vi "Main.vi"() -> ()   [LabVIEW 2018] (continued)
            n721 = Match Pattern(string=w6025, regular expression=w6022) -> (before substring=→"ST60 Sleeve 5020302":string)  [unwired: 1 in, 3 out]
            n722 = Match Pattern(string=w6024, regular expression=w6022) -> (before substring=→"ST60 Eclip 5018568":string)  [unwired: 1 in, 3 out]
            n723 = Match Pattern(string=w6023, regular expression=w6022) -> (before substring=→"ST70 Shaft Seal 5024366":string)  [unwired: 1 in, 3 out]
          }
        }
      }
      n724 = while {
        shift-right: [w4267] -> _
        shift-left: cluster{"Data":string[], "State":T1} {"Data"=[], "State"=enum."PLC通讯初始化"} ("元素") -> [w4268]
        shift-right: [w4276] -> _
        shift-left: w124 -> [w4273]
        shift-right: [w4277] -> _
        shift-left: _ -> [w4274]
        tunnel: w125 -> [w4269]
        tunnel: w123 -> [w4264]
        shift-right: [w4262] -> _
        shift-left: _ -> [w4263]
        tunnel: w122 -> [_]
        stop <- w4265 stop-if-true
        # "OP30"
        n725 = local read "退出"() -> (w4272:bool)
        n726 = Wait (ms)(milliseconds to wait=u32 20 ("等待时间（毫秒）")) -> ()  [unwired: 1 out]
        n727 = call "状态判断.vi"("error IO"=w4273, "退出？"=w4272, "簇 输入"=w4268, "队列输入"=w4269) -> ("簇"=w4271:cluster{"Data":string[], "State":T1})  [unwired: 6 in, 1 out]
        n728 = Unbundle By Name(w4271) -> ("Data"=w4266:string[], "State"=w4270:T1)
        "30_State" <- w4270
        n729 = case shown="\"读数据保存请求2\"" w4270 {
          tunnel: [w4287 w4326 w4346 w4377 w4398 w4450 w4470 w4516 w4529 w4544 w4564 w4609 w4628 w4682 w4688 w4752 w4779 w4795 refnum<k5> refnum ("TCP") refnum<k5> refnum ("TCP") w4814] -> w4277
          tunnel: [w4288 errorcluster {"status"=FALSE, "code"=0, "source"=""} ("error out") w4345 w4373 w4397 errorcluster {"status"=FALSE, "code"=0, "source"=""} ("error out") w4469 w4496 w4530 errorcluster {"status"=FALSE, "code"=0, "source"=""} ("error out") w4565 w4606 w4627 errorcluster {"status"=FALSE, "code"=0, "source"=""} ("error out") w4687 w4748 w4780 errorcluster {"status"=FALSE, "code"=0, "source"=""} ("error out") errorcluster {"status"=FALSE, "code"=0, "source"=""} ("error out") w4808 w4815] -> w4276
          tunnel: w4274 -> [_ w4326 w4347 w4378 w4399 w4450 w4471 w4498 w4532 w4544 w4550 w4611 w4632 w4682 w4690 w4742 w4783 w4795 w4802 w4809 w4826]
          tunnel: w4269 -> [w4317 _ w4328 _ _ _ w4451 _ _ _ w4562 _ _ _ w4686 _ _ _ w4798 w4810 _]
          tunnel: [cluster{"Data":string[], "State":T1} {"Data"=[], "State"=enum."读扫码请求"} ("元素") cluster{"Data":string[], "State":T1} {"Data"=[], "State"=enum."读扫码请求"} ("元素") w4335 cluster{"Data":string[], "State":T1} {"Data"=[], "State"=enum."读数据保存请求"} ("元素") cluster{"Data":string[], "State":T1} {"Data"=[], "State"=enum."读数据保存请求"} ("元素") cluster{"Data":string[], "State":T1} {"Data"=[], "State"=enum."读数据保存请求"} ("元素") w4459 cluster{"Data":string[], "State":T1} {"Data"=[], "State"=enum."读扫码请求2"} ("元素") cluster{"Data":string[], "State":T1} {"Data"=[], "State"=enum."读扫码请求2"} ("元素") cluster{"Data":string[], "State":T1} {"Data"=[], "State"=enum."读扫码请求2"} ("元素") w4563 cluster{"Data":string[], "State":T1} {"Data"=[], "State"=enum."读数据保存请求2"} ("元素") cluster{"Data":string[], "State":T1} {"Data"=[], "State"=enum."读数据保存请求2"} ("元素") cluster{"Data":string[], "State":T1} {"Data"=[], "State"=enum."读数据保存请求2"} ("元素") w4684 cluster{"Data":string[], "State":T1} {"Data"=[], "State"=enum."看门狗"} ("元素") cluster{"Data":string[], "State":T1} {"Data"=[], "State"=enum."看门狗"} ("元素") cluster{"Data":string[], "State":T1} {"Data"=[], "State"=enum."看门狗"} ("元素") cluster{"Data":string[], "State":T1} {"Data"=[], "State"=enum."PLC通讯初始化"} ("元素") cluster{"Data":string[], "State":T1} {"Data"=[], "State"=enum."退出"} ("元素") cluster{"Data":string[], "State":T1} {"Data"=[], "State"=enum."读扫码请求"} ("元素")] -> w4267
          tunnel: w4266 -> [_ _ _ _ w4396 _ _ _ w4531 _ _ _ w4631 _ _ _ w4781 _ _ _ _]
          tunnel: [FALSE FALSE FALSE FALSE FALSE FALSE FALSE FALSE FALSE FALSE FALSE FALSE FALSE FALSE FALSE FALSE FALSE FALSE FALSE TRUE FALSE] -> w4265
          tunnel: w4264 -> [_ _ _ _ _ _ _ w4508 _ _ _ _ _ _ _ _ _ _ w4799 w4811 _]
          tunnel: w4263 -> [_ w4322 w4329 w4374 w4394 w4446 w4452 w4499 w4526 w4540 w4549 w4610 w4633 w4683 w4689 w4750 w4782 w4796 w4797 w4806 w4819]
          tunnel: [T8 {"扫码2超时"="999", "扫码1超时"="999", "数据保存1超时"="999", "看门狗"="0", "数据保存2超时"="999"} w4322 w4329 w4374 w4393 w4446 w4452 w4499 w4524 w4540 w4548 w4610 w4626 w4683 w4689 w4750 w4777 w4796 w4797 w4806 w4818] -> w4262
          frame "PLC通讯初始化", Default {
            w4301 = u16 0 items=["byte", "word", "Dword"] ("数据类型")
            w4305 = u8 132 items=["I/O (P)"=128, "Input (I)"=129, "Output (Q)"=130, "Bit Memory (M)"=131, "Data (DB)"=132, "Instance Data (DI)"=133, "Local Data (L)"=134, "Predecessor Local Data (VL)"=135] ("寄存器类型")
            w4296 = u16 0 items=["byte", "word", "Dword"] ("数据类型")
            w4292 = u8 132 items=["I/O (P)"=128, "Input (I)"=129, "Output (Q)"=130, "Bit Memory (M)"=131, "Data (DB)"=132, "Instance Data (DI)"=133, "Local Data (L)"=134, "Predecessor Local Data (VL)"=135] ("寄存器类型")
            w4320 = u8 0 items=["S7-1200.200.200SMART"=0, "S7-300"=2, "S7-400"=3] ("PLC 系列")
            n730 = Enqueue Element(queue=w4317, element=cluster{"Data":string[], "State":T1} {"Data"=["999"], "State"=enum."扫码回复"} ("元素")) -> (queue out=w4313:refnum<queue>, error out=w4312:errorcluster)  [unwired: 2 in, 1 out]
            n731 = call "S7_Open.vi"("IP 地址"="192.168.0.30", "PLC 系列"=w4320, "超时（MS）"=100) -> ("TCP"=w4291:refnum<k5>, "error out"=w4290:errorcluster)  [unwired: 10 in, 1 out]
            n732 = Enqueue Element(queue=w4313, element=cluster{"Data":string[], "State":T1} {"Data"=["999"], "State"=enum."扫码回复2"} ("元素"), error in (no error)=w4312) -> (queue out=w4311:refnum<queue>, error out=w4310:errorcluster)  [unwired: 1 in, 1 out]
            n733 = Unbundle By Name(w4290) -> ("status"=→"ST30通讯状态":bool)
            n734 = call "S7_Read.vi"("TCP"=w4291, "DB #"=u16 20, "读取长度"=u16 17, "寄存器类型"=w4292, "起始地址"=u32 24, "数据类型"=w4296, "error in"=w4290) -> ("TCP"=w4306:refnum<k5>, "数据"=w4297:u32[], "error out"=w4289:errorcluster)  [unwired: 5 in, 1 out]
            n735 = Enqueue Element(queue=w4311, element=cluster{"Data":string[], "State":T1} {"Data"=["999"], "State"=enum."数据保存回复"} ("元素"), error in (no error)=w4310) -> (queue out=w4285:refnum<queue>, error out=w4284:errorcluster)  [unwired: 1 in, 1 out]
            n736 = To Unsigned Word Integer(number=w4297) -> (unsigned 16bit integer=w4298:u16[])
            n737 = call "还原为字符串.vi"("输入数组"=w4298) -> ("字符串"=w4282:string)  [unwired: 9 in, 1 out]
            n738 = Match Pattern(string=w4282, regular expression=" " ("正则表达式")) -> (before substring=w4281:string)  [unwired: 1 in, 3 out]
            n739 = local write "301 二维码"(w4281) -> ()
            n740 = Enqueue Element(queue=w4285, element=cluster{"Data":string[], "State":T1} {"Data"=["999"], "State"=enum."数据保存回复2"} ("元素"), error in (no error)=w4284) -> ()  [unwired: 1 in, 3 out]
            n741 = call "S7_Read.vi"("TCP"=w4306, "DB #"=u16 20, "读取长度"=u16 17, "寄存器类型"=w4305, "起始地址"=u32 42, "数据类型"=w4301, "error in"=w4289) -> ("TCP"=w4287:refnum<k5>, "数据"=w4300:u32[], "error out"=w4288:errorcluster)  [unwired: 5 in, 1 out]
            n742 = To Unsigned Word Integer(number=w4300) -> (unsigned 16bit integer=w4299:u16[])
            n743 = call "还原为字符串.vi"("输入数组"=w4299) -> ("字符串"=w4279:string)  [unwired: 9 in, 1 out]
            n744 = Match Pattern(string=w4279, regular expression=" " ("正则表达式")) -> (before substring=w4278:string)  [unwired: 1 in, 3 out]
            n745 = local write "302 二维码"(w4278) -> ()
          }
          frame "---------------" {
          }
          frame "读扫码请求" {
            w4355 = u16 0 items=["byte", "word", "Dword"] ("数据类型")
            w4357 = u8 132 items=["I/O (P)"=128, "Input (I)"=129, "Output (Q)"=130, "Bit Memory (M)"=131, "Data (DB)"=132, "Instance Data (DI)"=133, "Local Data (L)"=134, "Predecessor Local Data (VL)"=135] ("寄存器类型")
            n746 = call "S7_Read.vi"("TCP"=w4347, "DB #"=u16 20, "读取长度"=u16 1, "寄存器类型"=w4357, "起始地址"=u32 0, "数据类型"=w4355) -> ("TCP"=w4346:refnum<k5>, "数据"=w4352:u32[], "error out"=w4345:errorcluster)  [unwired: 6 in, 1 out]
            n747 = Index Array(array=w4352, index=0 ("索引")) -> (element=w4350:u32)
            n748 = Number To Boolean Array(number=w4350) -> (Boolean array=w4349:bool[])
            n749 = Index Array(array=w4349, index=0 ("索引")) -> (element=w4327:bool)
            "ST301扫码请求" <- w4327
            n750 = Unbundle By Name(w4329) -> ("扫码1超时"=w4330:string)
            n751 = Not Equal?(x=w4330, y="999") -> (x != y?=w4332:bool)
            n752 = Not(x=w4332) -> (.not. x?=w4333:bool)
            n753 = call <vilib>:"Boolean Crossing PtByPt.vi"("direction"=enum16{"either", "false-true", "true-false"}."false-true", "input"=w4327) -> ("crossing"=w4341:bool)  [unwired: 1 in]
            n754 = call <vilib>:"Boolean Crossing PtByPt.vi"("direction"=enum16{"either", "false-true", "true-false"}."true-false", "input"=w4327) -> ("crossing"=w4340:bool)  [unwired: 1 in]
            n755 = call "已用时间7"("Reset"=w4333) -> ("Time has Elapsed"=w4334:bool)  [unwired: 11 in, 7 out]
            n756 = Insert Into Array(array=bool[] [] ("数组"), index=0 ("索引"), new element #1=w4341, new element #2=w4340) -> (w4337:bool[])
            n757 = Boolean Array To Number(Boolean array=w4337) -> (number=w4336:u32)
            n758 = case shown="0, 默认" w4336 {
              tunnel: [cluster{"Data":string[], "State":T1} {"Data"=[], "State"=enum."读数据保存请求"} ("元素") w4363 w4366] -> w4335
              tunnel: w4328 -> [_ w4364 w4367]
              frame 0, Default {
              }
              frame 1 {
                w4363 = cluster{"Data":string[], "State":T1} {"Data"=[], "State"=enum."读二维码"} ("元素")
                n759 = Enqueue Element(queue=w4364, element=w4363, timeout in ms (-1)=10 ("超时毫秒(-1)")) -> ()  [unwired: 1 in, 3 out]
              }
              frame 2 {
                w4366 = cluster{"Data":string[], "State":T1} {"Data"=["999"], "State"=enum."扫码回复"} ("元素")
                n760 = Enqueue Element(queue=w4367, element=w4366, timeout in ms (-1)=10 ("超时毫秒(-1)")) -> ()  [unwired: 1 in, 3 out]
              }
            }
            n761 = case shown="真" w4334 {
              tunnel: w4328 -> [_ w4359]
              frame False {
              }
              frame True {
                n762 = Enqueue Element(queue=w4359, element=cluster{"Data":string[], "State":T1} {"Data"=["999"], "State"=enum."扫码回复"} ("元素"), timeout in ms (-1)=10 ("超时毫秒(-1)")) -> ()  [unwired: 1 in, 3 out]
              }
            }
          }
          frame "读二维码" {
            w4383 = u16 0 items=["byte", "word", "Dword"] ("数据类型")
            w4379 = u8 132 items=["I/O (P)"=128, "Input (I)"=129, "Output (Q)"=130, "Bit Memory (M)"=131, "Data (DB)"=132, "Instance Data (DI)"=133, "Local Data (L)"=134, "Predecessor Local Data (VL)"=135] ("寄存器类型")
            n763 = call "S7_Read.vi"("TCP"=w4378, "DB #"=u16 20, "读取长度"=u16 17, "寄存器类型"=w4379, "起始地址"=u32 24, "数据类型"=w4383) -> ("TCP"=w4377:refnum<k5>, "数据"=w4384:u32[], "error out"=w4386:errorcluster)  [unwired: 6 in, 1 out]
            n764 = To Unsigned Word Integer(number=w4384) -> (unsigned 16bit integer=w4385:u16[])
            n765 = call "还原为字符串.vi"("error in (no error)"=w4386, "输入数组"=w4385) -> ("error out"=w4370:errorcluster, "字符串"=w4371:string)  [unwired: 8 in]
            n766 = Match Pattern(string=w4371, regular expression=" " ("正则表达式")) -> (before substring=w4368:string)  [unwired: 1 in, 3 out]
            n767 = flat-sequence {
              tunnel: w4370 -> [w4388]
              tunnel: [w4388] -> w4369
              tunnel: w4368 -> [w4387]
              tunnel: [w4390] -> w4373
              tunnel: w4369 -> [w4389]
              frame #0 {
                "301 二维码" <- w4387
              }
              frame #1 {
                n768 = property on="ST301扫码请求 (事件)" class="Bool (严格)"(error in=w4389, "Val(Sgnl)"=TRUE ("值(信号)")) -> (error out=w4390:errorcluster)  [unwired: 1 in, 1 out]
              }
            }
          }
          frame "扫码回复" {
            n769 = Array Size(array=w4396) -> (size(s)=w4395:i32)
            n770 = case shown="1" w4395 {
              tunnel: w4399 -> [w4414 w4437]
              tunnel: [w4405 w4439] -> w4398
              tunnel: [w4404 w4438] -> w4397
              tunnel: w4396 -> [w4403 w4436]
              tunnel: [w4402 w4434] -> w4392
              frame 3, Default {
                w4417 = u8 132 items=["I/O (P)"=128, "Input (I)"=129, "Output (Q)"=130, "Bit Memory (M)"=131, "Data (DB)"=132, "Instance Data (DI)"=133, "Local Data (L)"=134, "Predecessor Local Data (VL)"=135] ("寄存器类型")
                w4416 = u16 1 items=["byte", "word", "Dword"] ("数据类型")
                w4424 = u8 132 items=["I/O (P)"=128, "Input (I)"=129, "Output (Q)"=130, "Bit Memory (M)"=131, "Data (DB)"=132, "Instance Data (DI)"=133, "Local Data (L)"=134, "Predecessor Local Data (VL)"=135] ("寄存器类型")
                w4425 = u16 1 items=["byte", "word", "Dword"] ("数据类型")
                w4430 = u8 132 items=["I/O (P)"=128, "Input (I)"=129, "Output (Q)"=130, "Bit Memory (M)"=131, "Data (DB)"=132, "Instance Data (DI)"=133, "Local Data (L)"=134, "Predecessor Local Data (VL)"=135] ("寄存器类型")
                w4429 = u16 1 items=["byte", "word", "Dword"] ("数据类型")
                n771 = Index Array(array=w4403) -> (element #1=w4402:string, element #2=w4410:string, element #3=w4409:string)  [unwired: 3 in]
                n772 = Equal?(x=w4409, y="OK") -> (x = y?=w4407:bool)
                n773 = Decimal String To Number(string=w4410, default (0L)=u32 0 ("默认(0 I32)")) -> (number=w4411:u32)  [unwired: 1 in, 1 out]
                n774 = case shown="真" w4407 {
                  tunnel: [u32 2 ("写入数据") u32 1 ("写入数据")] -> w4406
                  frame False {
                  }
                  frame True {
                  }
                }
                n775 = call "S7_Write.vi"("TCP"=w4414, "寄存器类型"=w4430, "DB #"=u16 20, "写入地址"=u32 8, "数据类型"=w4429, "写入数据"=w4411) -> ("TCP"=w4421:refnum<k5>, "error out"=w4422:errorcluster)  [unwired: 7 in, 1 out]
                n776 = call "S7_Write.vi"("TCP"=w4421, "寄存器类型"=w4424, "DB #"=u16 20, "写入地址"=u32 10, "数据类型"=w4425, "写入数据"=w4406, "error in"=w4422) -> ("TCP"=w4413:refnum<k5>, "error out"=w4412:errorcluster)  [unwired: 6 in, 1 out]
                n777 = Decimal String To Number(string=w4402, default (0L)=u32 0 ("默认(0 I32)")) -> (number=w4420:u32)  [unwired: 1 in, 1 out]
                n778 = call "S7_Write.vi"("TCP"=w4413, "寄存器类型"=w4417, "DB #"=u16 20, "写入地址"=u32 2, "数据类型"=w4416, "写入数据"=w4420, "error in"=w4412) -> ("TCP"=w4405:refnum<k5>, "error out"=w4404:errorcluster)  [unwired: 6 in, 1 out]
              }
              frame 1 {
                w4442 = u8 132 items=["I/O (P)"=128, "Input (I)"=129, "Output (Q)"=130, "Bit Memory (M)"=131, "Data (DB)"=132, "Instance Data (DI)"=133, "Local Data (L)"=134, "Predecessor Local Data (VL)"=135] ("寄存器类型")
                w4441 = u16 1 items=["byte", "word", "Dword"] ("数据类型")
                n779 = Index Array(array=w4436, index=0 ("索引")) -> (element=w4434:string)
                n780 = Decimal String To Number(string=w4434, default (0L)=u32 0 ("默认(0 I32)")) -> (number=w4445:u32)  [unwired: 1 in, 1 out]
                n781 = call "S7_Write.vi"("TCP"=w4437, "寄存器类型"=w4442, "DB #"=u16 20, "写入地址"=u32 2, "数据类型"=w4441, "写入数据"=w4445) -> ("TCP"=w4439:refnum<k5>, "error out"=w4438:errorcluster)  [unwired: 7 in, 1 out]
              }
            }
            "扫码请求回复301" <- w4392
            n782 = Bundle By Name(cluster=w4394, "扫码1超时"=w4392) -> (w4393:T8)
          }
          frame "-------------" {
          }
          frame "读数据保存请求" {
            w4479 = u16 0 items=["byte", "word", "Dword"] ("数据类型")
            w4481 = u8 132 items=["I/O (P)"=128, "Input (I)"=129, "Output (Q)"=130, "Bit Memory (M)"=131, "Data (DB)"=132, "Instance Data (DI)"=133, "Local Data (L)"=134, "Predecessor Local Data (VL)"=135] ("寄存器类型")
            n783 = call "S7_Read.vi"("TCP"=w4471, "DB #"=u16 20, "读取长度"=u16 1, "寄存器类型"=w4481, "起始地址"=u32 0, "数据类型"=w4479) -> ("TCP"=w4470:refnum<k5>, "数据"=w4476:u32[], "error out"=w4469:errorcluster)  [unwired: 6 in, 1 out]
            n784 = Index Array(array=w4476, index=0 ("索引")) -> (element=w4474:u32)
            n785 = Number To Boolean Array(number=w4474) -> (Boolean array=w4473:bool[])
            n786 = Unbundle By Name(w4452) -> ("数据保存1超时"=w4453:string)
            n787 = Index Array(array=w4473, index=1 ("索引")) -> (element=w4458:bool)
            "ST301数据读取" <- w4458
            n788 = Not Equal?(x=w4453, y="999") -> (x != y?=w4455:bool)
            n789 = Not(x=w4455) -> (.not. x?=w4456:bool)
            n790 = call <vilib>:"Boolean Crossing PtByPt.vi"("direction"=enum16{"either", "false-true", "true-false"}."false-true", "input"=w4458) -> ("crossing"=w4462:bool)  [unwired: 1 in]
            n791 = call <vilib>:"Boolean Crossing PtByPt.vi"("direction"=enum16{"either", "false-true", "true-false"}."true-false", "input"=w4458) -> ("crossing"=w4463:bool)  [unwired: 1 in]
            n792 = call "已用时间8"("Reset"=w4456) -> ("Time has Elapsed"=w4457:bool)  [unwired: 11 in, 7 out]
            n793 = Insert Into Array(array=bool[] [] ("数组"), index=0 ("索引"), new element #1=w4462, new element #2=w4463) -> (w4466:bool[])
            n794 = Boolean Array To Number(Boolean array=w4466) -> (number=w4467:u32)
            n795 = case shown="2" w4467 {
              tunnel: [cluster{"Data":string[], "State":T1} {"Data"=[], "State"=enum."读扫码请求2"} ("元素") w4487 w4489] -> w4459
              tunnel: w4451 -> [_ w4488 w4490]
              frame 0, Default {
              }
              frame 1 {
                w4487 = cluster{"Data":string[], "State":T1} {"Data"=[], "State"=enum."读数据"} ("元素")
                n796 = Enqueue Element(queue=w4488, element=w4487, timeout in ms (-1)=10 ("超时毫秒(-1)")) -> ()  [unwired: 1 in, 3 out]
              }
              frame 2 {
                w4489 = cluster{"Data":string[], "State":T1} {"Data"=["999"], "State"=enum."数据保存回复"} ("元素")
                n797 = Enqueue Element(queue=w4490, element=w4489, timeout in ms (-1)=10 ("超时毫秒(-1)")) -> ()  [unwired: 1 in, 3 out]
              }
            }
            n798 = case shown="真" w4457 {
              tunnel: w4451 -> [_ w4483]
              frame False {
              }
              frame True {
                n799 = Enqueue Element(queue=w4483, element=cluster{"Data":string[], "State":T1} {"Data"=["999"], "State"=enum."数据保存回复"} ("元素"), timeout in ms (-1)=10 ("超时毫秒(-1)")) -> ()  [unwired: 1 in, 3 out]
              }
            }
          }
          frame "读数据" {
            w4517 = u16 1 items=["byte", "word", "Dword"] ("数据类型")
            w4521 = u8 132 items=["I/O (P)"=128, "Input (I)"=129, "Output (Q)"=130, "Bit Memory (M)"=131, "Data (DB)"=132, "Instance Data (DI)"=133, "Local Data (L)"=134, "Predecessor Local Data (VL)"=135] ("寄存器类型")
            n800 = call "S7_Read.vi"("TCP"=w4498, "DB #"=u16 20, "读取长度"=u16 1, "寄存器类型"=w4521, "起始地址"=u32 6, "数据类型"=w4517) -> ("TCP"=w4516:refnum<k5>, "数据"=w4513:u32[], "error out"=w4507:errorcluster)  [unwired: 6 in, 1 out]
            n801 = local read "ST301 Dowel Pin 5024533"() -> (w4493:string)
            n802 = local read "ST301 Dowel Pin 5020282"() -> (w4492:string)
            n803 = Index Array(array=w4513) -> (element=w4512:u32)  [unwired: 1 in]
            n804 = local read "ST301 Vane 5004737"() -> (w4494:string)
            n805 = Equal?(x=w4512, y=u32 1) -> (x = y?=w4510:bool)
            n806 = case shown="真" w4510 {
              tunnel: ["NG" "OK"] -> w4500
              frame False {
              }
              frame True {
              }
            }
            n807 = Format Date/Time String(time format string (%c)="%Y-%m-%d" ("时间格式字符串(%c)")) -> (date/time string=w4502:string)  [unwired: 2 in]
            n808 = Get Date/Time String() -> (time string=w4501:string)  [unwired: 3 in, 1 out]
            n809 = Insert Into Array(array=string[] [] ("数组"), index=0 ("索引"), new element #1="301" ("新元素/子数组"), new element #2=w4500, new element #3=w4502, new element #4=w4501, new element #5=w4500, new element #6=w4494, new element #7=w4493, new element #8=w4492) -> (w4509:string[])
            n810 = Enqueue Element(queue=w4508, element=w4509, error in (no error)=w4507) -> (error out=w4497:errorcluster)  [unwired: 1 in, 2 out]
            n811 = property on="ST301数据读取 (事件)" class="Bool (严格)"(error in=w4497, "Val(Sgnl)"=TRUE ("值(信号)")) -> (error out=w4496:errorcluster)  [unwired: 1 in, 1 out]
          }
          frame "数据保存回复" {
            w4537 = u8 132 items=["I/O (P)"=128, "Input (I)"=129, "Output (Q)"=130, "Bit Memory (M)"=131, "Data (DB)"=132, "Instance Data (DI)"=133, "Local Data (L)"=134, "Predecessor Local Data (VL)"=135] ("寄存器类型")
            w4538 = u16 1 items=["byte", "word", "Dword"] ("数据类型")
            n812 = Index Array(array=w4531, index=0 ("索引")) -> (element=w4525:string)
            "数据保存请求回复301" <- w4525
            n813 = Decimal String To Number(string=w4525, default (0L)=u32 0 ("默认(0 I32)")) -> (number=w4533:u32)  [unwired: 1 in, 1 out]
            n814 = call "S7_Write.vi"("TCP"=w4532, "寄存器类型"=w4537, "DB #"=u16 20, "写入地址"=u32 4, "数据类型"=w4538, "写入数据"=w4533) -> ("TCP"=w4529:refnum<k5>, "error out"=w4530:errorcluster)  [unwired: 7 in, 1 out]
            n815 = Bundle By Name(cluster=w4526, "数据保存1超时"=w4525) -> (w4524:T8)
          }
          frame "-----------------" {
          }
          frame "读扫码请求2" {
            w4558 = u8 132 items=["I/O (P)"=128, "Input (I)"=129, "Output (Q)"=130, "Bit Memory (M)"=131, "Data (DB)"=132, "Instance Data (DI)"=133, "Local Data (L)"=134, "Predecessor Local Data (VL)"=135] ("寄存器类型")
            w4557 = u16 1 items=["byte", "word", "Dword"] ("数据类型")
            w4566 = u16 0 items=["byte", "word", "Dword"] ("数据类型")
            w4568 = u8 132 items=["I/O (P)"=128, "Input (I)"=129, "Output (Q)"=130, "Bit Memory (M)"=131, "Data (DB)"=132, "Instance Data (DI)"=133, "Local Data (L)"=134, "Predecessor Local Data (VL)"=135] ("寄存器类型")
            n816 = Unbundle By Name(w4549) -> ("看门狗"=w4555:string)
            n817 = Decimal String To Number(string=w4555) -> (number=w4554:i32)  [unwired: 2 in, 1 out]
            n818 = Equal?(x=w4554, y=0) -> (x = y?=w4552:bool)
            n819 = case shown="假" w4552 {
              tunnel: [0 ("y") 1 ("y")] -> w4545
              frame False {
              }
              frame True {
              }
            }
            n820 = call "S7_Write.vi"("TCP"=w4550, "寄存器类型"=w4558, "DB #"=u16 20, "写入地址"=u32 22, "数据类型"=w4557, "写入数据"=w4545) -> ("TCP"=w4546:refnum<k5>, "error out"=w4547:errorcluster)  [unwired: 7 in, 1 out]
            n821 = Number To Decimal String(number=w4545) -> (decimal integer string=w4551:string)  [unwired: 1 in]
            n822 = local write "30"(w4545) -> ()
            n823 = Bundle By Name(cluster=w4549, "看门狗"=w4551) -> (w4548:T8)
            n824 = call "S7_Read.vi"("TCP"=w4546, "DB #"=u16 20, "读取长度"=u16 1, "寄存器类型"=w4568, "起始地址"=u32 0, "数据类型"=w4566, "error in"=w4547) -> ("TCP"=w4564:refnum<k5>, "数据"=w4588:u32[], "error out"=w4565:errorcluster)  [unwired: 5 in, 1 out]
            n825 = Index Array(array=w4588, index=0 ("索引")) -> (element=w4587:u32)
            n826 = Number To Boolean Array(number=w4587) -> (Boolean array=w4586:bool[])
            n827 = Index Array(array=w4586, index=2 ("索引")) -> (element=w4561:bool)
            "ST302扫码请求" <- w4561
            n828 = Unbundle By Name(w4548) -> ("扫码2超时"=w4578:string)
            n829 = Not Equal?(x=w4578, y="999") -> (x != y?=w4579:bool)
            n830 = Not(x=w4579) -> (.not. x?=w4580:bool)
            n831 = call <vilib>:"Boolean Crossing PtByPt.vi"("direction"=enum16{"either", "false-true", "true-false"}."false-true", "input"=w4561) -> ("crossing"=w4585:bool)  [unwired: 1 in]
            n832 = call <vilib>:"Boolean Crossing PtByPt.vi"("direction"=enum16{"either", "false-true", "true-false"}."true-false", "input"=w4561) -> ("crossing"=w4584:bool)  [unwired: 1 in]
            n833 = call "已用时间23"("Reset"=w4580) -> ("Time has Elapsed"=w4581:bool)  [unwired: 11 in, 7 out]
            n834 = Insert Into Array(array=bool[] [] ("数组"), index=0 ("索引"), new element #1=w4585, new element #2=w4584) -> (w4583:bool[])
            n835 = Boolean Array To Number(Boolean array=w4583) -> (number=w4582:u32)
            n836 = case shown="0, 默认" w4582 {
              tunnel: [cluster{"Data":string[], "State":T1} {"Data"=[], "State"=enum."读数据保存请求2"} ("元素") w4596 w4599] -> w4563
              tunnel: w4562 -> [_ w4597 w4600]
              frame 0, Default {
              }
              frame 1 {
                w4596 = cluster{"Data":string[], "State":T1} {"Data"=[], "State"=enum."读二维码2"} ("元素")
                n837 = Enqueue Element(queue=w4597, element=w4596, timeout in ms (-1)=10 ("超时毫秒(-1)")) -> ()  [unwired: 1 in, 3 out]
              }
              frame 2 {
                w4599 = cluster{"Data":string[], "State":T1} {"Data"=["999"], "State"=enum."扫码回复2"} ("元素")
                n838 = Enqueue Element(queue=w4600, element=w4599, timeout in ms (-1)=10 ("超时毫秒(-1)")) -> ()  [unwired: 1 in, 3 out]
              }
            }
            n839 = case shown="真" w4581 {
              tunnel: w4562 -> [_ w4592]
              frame False {
              }
              frame True {
                n840 = Enqueue Element(queue=w4592, element=cluster{"Data":string[], "State":T1} {"Data"=["999"], "State"=enum."扫码回复2"} ("元素"), timeout in ms (-1)=10 ("超时毫秒(-1)")) -> ()  [unwired: 1 in, 3 out]
              }
            }
          }
          frame "读二维码2" {
            w4612 = u16 0 items=["byte", "word", "Dword"] ("数据类型")
            w4614 = u8 132 items=["I/O (P)"=128, "Input (I)"=129, "Output (Q)"=130, "Bit Memory (M)"=131, "Data (DB)"=132, "Instance Data (DI)"=133, "Local Data (L)"=134, "Predecessor Local Data (VL)"=135] ("寄存器类型")
            n841 = call "S7_Read.vi"("TCP"=w4611, "DB #"=u16 20, "读取长度"=u16 17, "寄存器类型"=w4614, "起始地址"=u32 42, "数据类型"=w4612) -> ("TCP"=w4609:refnum<k5>, "数据"=w4617:u32[], "error out"=w4619:errorcluster)  [unwired: 6 in, 1 out]
            n842 = To Unsigned Word Integer(number=w4617) -> (unsigned 16bit integer=w4618:u16[])
            n843 = call "还原为字符串.vi"("error in (no error)"=w4619, "输入数组"=w4618) -> ("error out"=w4603:errorcluster, "字符串"=w4604:string)  [unwired: 8 in]
            n844 = Match Pattern(string=w4604, regular expression=" " ("正则表达式")) -> (before substring=w4601:string)  [unwired: 1 in, 3 out]
            n845 = flat-sequence {
              tunnel: w4603 -> [w4621]
              tunnel: [w4621] -> w4602
              tunnel: w4601 -> [w4620]
              tunnel: [w4623] -> w4606
              tunnel: w4602 -> [w4622]
              frame #0 {
                "302 二维码" <- w4620
              }
              frame #1 {
                n846 = property on="ST302扫码请求 (事件)" class="Bool (严格)"(error in=w4622, "Val(Sgnl)"=TRUE ("值(信号)")) -> (error out=w4623:errorcluster)  [unwired: 1 in, 1 out]
              }
            }
          }
          frame "扫码回复2" {
            n847 = Array Size(array=w4631) -> (size(s)=w4634:i32)
            n848 = case shown="1" w4634 {
              tunnel: w4632 -> [w4647 w4670]
              tunnel: [w4638 w4672] -> w4628
              tunnel: [w4637 w4671] -> w4627
              tunnel: w4631 -> [w4636 w4669]
              tunnel: [w4635 w4667] -> w4629
              frame 3, Default {
                w4650 = u8 132 items=["I/O (P)"=128, "Input (I)"=129, "Output (Q)"=130, "Bit Memory (M)"=131, "Data (DB)"=132, "Instance Data (DI)"=133, "Local Data (L)"=134, "Predecessor Local Data (VL)"=135] ("寄存器类型")
                w4649 = u16 1 items=["byte", "word", "Dword"] ("数据类型")
                w4657 = u8 132 items=["I/O (P)"=128, "Input (I)"=129, "Output (Q)"=130, "Bit Memory (M)"=131, "Data (DB)"=132, "Instance Data (DI)"=133, "Local Data (L)"=134, "Predecessor Local Data (VL)"=135] ("寄存器类型")
                w4658 = u16 1 items=["byte", "word", "Dword"] ("数据类型")
                w4663 = u8 132 items=["I/O (P)"=128, "Input (I)"=129, "Output (Q)"=130, "Bit Memory (M)"=131, "Data (DB)"=132, "Instance Data (DI)"=133, "Local Data (L)"=134, "Predecessor Local Data (VL)"=135] ("寄存器类型")
                w4662 = u16 1 items=["byte", "word", "Dword"] ("数据类型")
                n849 = Index Array(array=w4636) -> (element #1=w4635:string, element #2=w4643:string, element #3=w4642:string)  [unwired: 3 in]
                n850 = Equal?(x=w4642, y="OK") -> (x = y?=w4640:bool)
                n851 = Decimal String To Number(string=w4643, default (0L)=u32 0 ("默认(0 I32)")) -> (number=w4644:u32)  [unwired: 1 in, 1 out]
                n852 = case shown="真" w4640 {
                  tunnel: [u32 2 ("写入数据") u32 1 ("写入数据")] -> w4639
                  frame False {
                  }
                  frame True {
                  }
                }
                n853 = call "S7_Write.vi"("TCP"=w4647, "寄存器类型"=w4663, "DB #"=u16 20, "写入地址"=u32 18, "数据类型"=w4662, "写入数据"=w4644) -> ("TCP"=w4654:refnum<k5>, "error out"=w4655:errorcluster)  [unwired: 7 in, 1 out]
                n854 = call "S7_Write.vi"("TCP"=w4654, "寄存器类型"=w4657, "DB #"=u16 20, "写入地址"=u32 20, "数据类型"=w4658, "写入数据"=w4639, "error in"=w4655) -> ("TCP"=w4646:refnum<k5>, "error out"=w4645:errorcluster)  [unwired: 6 in, 1 out]
                n855 = Decimal String To Number(string=w4635, default (0L)=u32 0 ("默认(0 I32)")) -> (number=w4653:u32)  [unwired: 1 in, 1 out]
                n856 = call "S7_Write.vi"("TCP"=w4646, "寄存器类型"=w4650, "DB #"=u16 20, "写入地址"=u32 14, "数据类型"=w4649, "写入数据"=w4653, "error in"=w4645) -> ("TCP"=w4638:refnum<k5>, "error out"=w4637:errorcluster)  [unwired: 6 in, 1 out]
              }
              frame 1 {
                w4675 = u8 132 items=["I/O (P)"=128, "Input (I)"=129, "Output (Q)"=130, "Bit Memory (M)"=131, "Data (DB)"=132, "Instance Data (DI)"=133, "Local Data (L)"=134, "Predecessor Local Data (VL)"=135] ("寄存器类型")
                w4674 = u16 1 items=["byte", "word", "Dword"] ("数据类型")
                n857 = Index Array(array=w4669, index=0 ("索引")) -> (element=w4667:string)
                n858 = Decimal String To Number(string=w4667, default (0L)=u32 0 ("默认(0 I32)")) -> (number=w4678:u32)  [unwired: 1 in, 1 out]
                n859 = call "S7_Write.vi"("TCP"=w4670, "寄存器类型"=w4675, "DB #"=u16 20, "写入地址"=u32 14, "数据类型"=w4674, "写入数据"=w4678) -> ("TCP"=w4672:refnum<k5>, "error out"=w4671:errorcluster)  [unwired: 7 in, 1 out]
              }
            }
            "扫码请求回复302" <- w4629
            n860 = Bundle By Name(cluster=w4633, "扫码2超时"=w4629) -> (w4626:T8)
          }
          frame "-- --------------" {
          }
          frame "读数据保存请求2" {
            w4691 = u16 0 items=["byte", "word", "Dword"] ("数据类型")
            w4693 = u8 132 items=["I/O (P)"=128, "Input (I)"=129, "Output (Q)"=130, "Bit Memory (M)"=131, "Data (DB)"=132, "Instance Data (DI)"=133, "Local Data (L)"=134, "Predecessor Local Data (VL)"=135] ("寄存器类型")
            n861 = call "S7_Read.vi"("TCP"=w4690, "DB #"=u16 20, "读取长度"=u16 1, "寄存器类型"=w4693, "起始地址"=u32 0, "数据类型"=w4691) -> ("TCP"=w4688:refnum<k5>, "数据"=w4714:u32[], "error out"=w4687:errorcluster)  [unwired: 6 in, 1 out]
            n862 = Index Array(array=w4714, index=0 ("索引")) -> (element=w4713:u32)
            n863 = Number To Boolean Array(number=w4713) -> (Boolean array=w4712:bool[])
            n864 = Unbundle By Name(w4689) -> ("数据保存2超时"=w4703:string)
            n865 = Index Array(array=w4712, index=3 ("索引")) -> (element=w4707:bool)
            "ST302数据读取" <- w4707
            n866 = Not Equal?(x=w4703, y="999") -> (x != y?=w4704:bool)
            n867 = Not(x=w4704) -> (.not. x?=w4705:bool)
            n868 = call <vilib>:"Boolean Crossing PtByPt.vi"("direction"=enum16{"either", "false-true", "true-false"}."false-true", "input"=w4707) -> ("crossing"=w4708:bool)  [unwired: 1 in]
            n869 = call <vilib>:"Boolean Crossing PtByPt.vi"("direction"=enum16{"either", "false-true", "true-false"}."true-false", "input"=w4707) -> ("crossing"=w4709:bool)  [unwired: 1 in]
            n870 = call "已用时间24"("Reset"=w4705) -> ("Time has Elapsed"=w4706:bool)  [unwired: 11 in, 7 out]
            n871 = Insert Into Array(array=bool[] [] ("数组"), index=0 ("索引"), new element #1=w4708, new element #2=w4709) -> (w4710:bool[])
            n872 = Boolean Array To Number(Boolean array=w4710) -> (number=w4711:u32)
            n873 = case shown="1" w4711 {
              tunnel: [cluster{"Data":string[], "State":T1} {"Data"=[], "State"=enum."看门狗"} ("元素") w4720 w4722] -> w4684
              tunnel: w4686 -> [_ w4721 w4723]
              frame 0, Default {
              }
              frame 1 {
                w4720 = cluster{"Data":string[], "State":T1} {"Data"=[], "State"=enum."读数据2"} ("元素")
                n874 = Enqueue Element(queue=w4721, element=w4720, timeout in ms (-1)=10 ("超时毫秒(-1)")) -> ()  [unwired: 1 in, 3 out]
              }
              frame 2 {
                w4722 = cluster{"Data":string[], "State":T1} {"Data"=["999"], "State"=enum."数据保存回复2"} ("元素")
                n875 = Enqueue Element(queue=w4723, element=w4722, timeout in ms (-1)=10 ("超时毫秒(-1)")) -> ()  [unwired: 1 in, 3 out]
              }
            }
            n876 = case shown="真" w4706 {
              tunnel: w4686 -> [_ w4716]
              frame False {
              }
              frame True {
                n877 = Enqueue Element(queue=w4716, element=cluster{"Data":string[], "State":T1} {"Data"=["999"], "State"=enum."数据保存回复2"} ("元素"), timeout in ms (-1)=10 ("超时毫秒(-1)")) -> ()  [unwired: 1 in, 3 out]
              }
            }
          }
          frame "读数据2" {
            w4732 = i16 4 ("精度(6)")
            w4747 = u16 2 items=["byte", "word", "Dword"] ("数据类型")
            w4745 = u8 132 items=["I/O (P)"=128, "Input (I)"=129, "Output (Q)"=130, "Bit Memory (M)"=131, "Data (DB)"=132, "Instance Data (DI)"=133, "Local Data (L)"=134, "Predecessor Local Data (VL)"=135] ("寄存器类型")
            w4753 = u16 1 items=["byte", "word", "Dword"] ("数据类型")
            w4755 = u8 132 items=["I/O (P)"=128, "Input (I)"=129, "Output (Q)"=130, "Bit Memory (M)"=131, "Data (DB)"=132, "Instance Data (DI)"=133, "Local Data (L)"=134, "Predecessor Local Data (VL)"=135] ("寄存器类型")
            n878 = call "S7_Read.vi"("TCP"=w4742, "DB #"=u16 20, "读取长度"=u16 4, "寄存器类型"=w4745, "起始地址"=u32 60, "数据类型"=w4747) -> ("TCP"=w4741:refnum<k5>, "数据"=w4739:u32[], "error out"=w4740:errorcluster)  [unwired: 6 in, 1 out]
            n879 = Divide(x=w4739, y=u32[] [10000, 10000, 10000, 10000]) -> (x/y=w4737:dbl[])
            n880 = Index Array(array=w4737) -> (element #1=w4736:dbl, element #2=w4735:dbl, element #3=w4734:dbl, element #4=w4733:dbl)  [unwired: 4 in]
            n881 = Number To Fractional String(number=w4736, precision (6)=w4732) -> (F-format string=w4731:string)  [unwired: 2 in]
            n882 = Number To Fractional String(number=w4735, precision (6)=w4732) -> (F-format string=w4730:string)  [unwired: 2 in]
            n883 = Number To Fractional String(number=w4734, precision (6)=w4732) -> (F-format string=w4729:string)  [unwired: 2 in]
            n884 = Number To Fractional String(number=w4733, precision (6)=w4732) -> (F-format string=w4728:string)  [unwired: 2 in]
            n885 = call "S7_Read.vi"("TCP"=w4741, "DB #"=u16 20, "读取长度"=u16 1, "寄存器类型"=w4755, "起始地址"=u32 12, "数据类型"=w4753, "error in"=w4740) -> ("TCP"=w4752:refnum<k5>, "数据"=w4768:u32[], "error out"=w4727:errorcluster)  [unwired: 5 in, 1 out]
            n886 = Index Array(array=w4768) -> (element=w4767:u32)  [unwired: 1 in]
            n887 = Equal?(x=w4767, y=u32 1) -> (x = y?=w4766:bool)
            n888 = case shown="真" w4766 {
              tunnel: ["NG" "OK"] -> w4763
              frame False {
              }
              frame True {
              }
            }
            n889 = Format Date/Time String(time format string (%c)="%Y-%m-%d" ("时间格式字符串(%c)")) -> (date/time string=w4765:string)  [unwired: 2 in]
            n890 = Get Date/Time String() -> (time string=w4764:string)  [unwired: 3 in, 1 out]
            n891 = Insert Into Array(array=string[] [] ("数组"), index=0 ("索引"), new element #1="302" ("新元素/子数组"), new element #2=w4763, new element #3=w4765, new element #4=w4764, new element #5=w4763, new element #6=w4731, new element #7=w4730, new element #8=w4729, new element #9=w4728) -> (w4725:string[])
            n892 = flat-sequence {
              tunnel: w4727 -> [w4770]
              tunnel: [w4770] -> w4726
              tunnel: w4725 -> [w4769]
              tunnel: [w4773] -> w4748
              tunnel: w4726 -> [w4771]
              frame #0 {
                "302读取数据" <- w4769
              }
              frame #1 {
                n893 = property on="ST302数据读取 (事件)" class="Bool (严格)"(error in=w4771, "Val(Sgnl)"=TRUE ("值(信号)")) -> (error out=w4773:errorcluster)  [unwired: 1 in, 1 out]
              }
            }
          }
          frame "数据保存回复2" {
            w4787 = u8 132 items=["I/O (P)"=128, "Input (I)"=129, "Output (Q)"=130, "Bit Memory (M)"=131, "Data (DB)"=132, "Instance Data (DI)"=133, "Local Data (L)"=134, "Predecessor Local Data (VL)"=135] ("寄存器类型")
            w4784 = u16 1 items=["byte", "word", "Dword"] ("数据类型")
            n894 = Index Array(array=w4781, index=0 ("索引")) -> (element=w4790:string)
            "数据保存请求回复302" <- w4790
            n895 = Decimal String To Number(string=w4790, default (0L)=u32 0 ("默认(0 I32)")) -> (number=w4791:u32)  [unwired: 1 in, 1 out]
            n896 = call "S7_Write.vi"("TCP"=w4783, "寄存器类型"=w4787, "DB #"=u16 20, "写入地址"=u32 16, "数据类型"=w4784, "写入数据"=w4791) -> ("TCP"=w4779:refnum<k5>, "error out"=w4780:errorcluster)  [unwired: 7 in, 1 out]
            n897 = Bundle By Name(cluster=w4782, "数据保存2超时"=w4790) -> (w4777:T8)
          }
          frame "------------" {
          }
          frame "错误" {
            n898 = Flush Queue(queue=w4799) -> ()  [unwired: 1 in, 3 out]
            n899 = Flush Queue(queue=w4798) -> ()  [unwired: 1 in, 3 out]
            n900 = call "S7_Close.vi"("TCP Connection Ref"=w4802) -> ("error out"=w4800:errorcluster)  [unwired: 10 in]
            n901 = call <vilib>:"Clear Errors.vi"("error in (no error)"=w4800) -> ()  [unwired: 5 in, 2 out]
          }
          frame "退出" {
            n902 = Release Queue(queue=w4811) -> ()  [unwired: 2 in, 3 out]
            n903 = Release Queue(queue=w4810) -> ()  [unwired: 2 in, 3 out]
            n904 = call "S7_Close.vi"("TCP Connection Ref"=w4809) -> ("error out"=w4808:errorcluster)  [unwired: 10 in]
          }
          frame "看门狗" {
            w4829 = u8 132 items=["I/O (P)"=128, "Input (I)"=129, "Output (Q)"=130, "Bit Memory (M)"=131, "Data (DB)"=132, "Instance Data (DI)"=133, "Local Data (L)"=134, "Predecessor Local Data (VL)"=135] ("寄存器类型")
            w4828 = u16 1 items=["byte", "word", "Dword"] ("数据类型")
            n905 = Unbundle By Name(w4819) -> ("看门狗"=w4825:string)
            n906 = Decimal String To Number(string=w4825) -> (number=w4824:i32)  [unwired: 2 in, 1 out]
            n907 = Equal?(x=w4824, y=0) -> (x = y?=w4822:bool)
            n908 = case shown="假" w4822 {
              tunnel: [0 ("y") 1 ("y")] -> w4821
              frame False {
              }
              frame True {
              }
            }
            "30" <- w4821
            n909 = call "S7_Write.vi"("TCP"=w4826, "寄存器类型"=w4829, "DB #"=u16 20, "写入地址"=u32 22, "数据类型"=w4828, "写入数据"=w4821) -> ("TCP"=w4817:refnum<k5>, "error out"=w4816:errorcluster)  [unwired: 7 in, 1 out]
            n910 = Number To Decimal String(number=w4821) -> (decimal integer string=w4820:string)  [unwired: 1 in]
            n911 = Bundle By Name(cluster=w4819, "看门狗"=w4820) -> (w4818:T8)
            n912 = disable-structure shown="启用" {
              disable-tunnel: w4817 -> [w4833 w4837]
              disable-tunnel: [w4833 w4840] -> w4814
              disable-tunnel: w4816 -> [w4834 w4838]
              disable-tunnel: [w4834 w4839] -> w4815
              frame Disabled {
              }
              frame Enabled {
                w4842 = u8 132 items=["I/O (P)"=128, "Input (I)"=129, "Output (Q)"=130, "Bit Memory (M)"=131, "Data (DB)"=132, "Instance Data (DI)"=133, "Local Data (L)"=134, "Predecessor Local Data (VL)"=135] ("寄存器类型")
                w4836 = u16 1 items=["byte", "word", "Dword"] ("数据类型")
                n913 = local read "80产品型号"() -> (w4835:u32)
                n914 = call "S7_Write.vi"("TCP"=w4837, "寄存器类型"=w4842, "DB #"=u16 20, "写入地址"=u32 76, "数据类型"=w4836, "写入数据"=w4835, "error in"=w4838) -> ("TCP"=w4840:refnum<k5>, "error out"=w4839:errorcluster)  [unwired: 6 in, 1 out]
              }
            }
          }
        }
      }
      n915 = while {
        shift-right: [w3398] -> _
        shift-left: cluster{"Data":string[], "State":T1} {"Data"=[], "State"=enum."PLC通讯初始化"} ("元素") -> [w3399]
        shift-right: [w3407] -> _
        shift-left: w119 -> [w3404]
        shift-right: [w3408] -> _
        shift-left: _ -> [w3405]
        tunnel: w120 -> [w3400]
        tunnel: w118 -> [w3395]
        shift-right: [w3394] -> _
        shift-left: _ -> [w3393]
        tunnel: w117 -> [_]
        stop <- w3396 stop-if-true
        # "OP40"
        n916 = local read "退出"() -> (w3403:bool)
        n917 = Wait (ms)(milliseconds to wait=u32 20 ("等待时间（毫秒）")) -> ()  [unwired: 1 out]
        n918 = call "状态判断.vi"("error IO"=w3404, "退出？"=w3403, "簇 输入"=w3399, "队列输入"=w3400) -> ("簇"=w3402:cluster{"Data":string[], "State":T1})  [unwired: 6 in, 1 out]
        n919 = Unbundle By Name(w3402) -> ("Data"=w3397:string[], "State"=w3401:T1)
        "40_State" <- w3401
        n920 = case shown="\"读二维码\"" w3401 {
          tunnel: [w3417 w3485 w3507 w3538 w3559 w3610 w3630 w3676 w3704 w3719 refnum<k5> refnum ("TCP") refnum<k5> refnum ("TCP") w3741 w3752 w3789 w3817 w3868 w3893 w3929 w3964 w3977 w3989 w4029 w4048 w4100 w4104 w4182 w4212 w4228 w4232] -> w3408
          tunnel: [w3416 errorcluster {"status"=FALSE, "code"=0, "source"=""} ("error out") w3506 w3534 w3558 errorcluster {"status"=FALSE, "code"=0, "source"=""} ("error out") w3629 w3670 w3705 errorcluster {"status"=FALSE, "code"=0, "source"=""} ("error out") errorcluster {"status"=FALSE, "code"=0, "source"=""} ("error out") w3731 errorcluster {"status"=FALSE, "code"=0, "source"=""} ("error out") w3751 w3784 w3816 errorcluster {"status"=FALSE, "code"=0, "source"=""} ("error out") w3892 w3926 w3963 errorcluster {"status"=FALSE, "code"=0, "source"=""} ("error out") w3988 w4025 w4047 errorcluster {"status"=FALSE, "code"=0, "source"=""} ("error out") w4106 w4179 w4211 errorcluster {"status"=FALSE, "code"=0, "source"=""} ("error out") w4230] -> w3407
          tunnel: w3405 -> [_ w3485 w3508 w3539 w3560 w3610 w3631 w3656 w3707 w3719 w3725 w3732 w3741 w3753 w3790 w3818 w3868 w3874 w3928 w3966 w3977 w3990 w4030 w4050 w4100 w4108 w4157 w4214 w4228 w4240]
          tunnel: w3400 -> [w3447 _ w3488 _ _ _ w3611 _ _ _ w3721 w3733 _ w3742 _ _ _ w3884 _ _ _ w3979 _ _ _ w4107 _ _ _ _]
          tunnel: [cluster{"Data":string[], "State":T1} {"Data"=[], "State"=enum."读扫码请求"} ("元素") cluster{"Data":string[], "State":T1} {"Data"=[], "State"=enum."读扫码请求"} ("元素") w3496 cluster{"Data":string[], "State":T1} {"Data"=[], "State"=enum."读数据保存请求"} ("元素") cluster{"Data":string[], "State":T1} {"Data"=[], "State"=enum."读数据保存请求"} ("元素") cluster{"Data":string[], "State":T1} {"Data"=[], "State"=enum."读数据保存请求"} ("元素") w3619 cluster{"Data":string[], "State":T1} {"Data"=[], "State"=enum."读扫码请求3"} ("元素") cluster{"Data":string[], "State":T1} {"Data"=[], "State"=enum."读扫码请求3"} ("元素") cluster{"Data":string[], "State":T1} {"Data"=[], "State"=enum."读扫码请求3"} ("元素") cluster{"Data":string[], "State":T1} {"Data"=[], "State"=enum."PLC通讯初始化"} ("元素") cluster{"Data":string[], "State":T1} {"Data"=[], "State"=enum."退出"} ("元素") cluster{"Data":string[], "State":T1} {"Data"=[], "State"=enum."读扫码请求3"} ("元素") w3750 cluster{"Data":string[], "State":T1} {"Data"=[], "State"=enum."读数据保存请求2"} ("元素") cluster{"Data":string[], "State":T1} {"Data"=[], "State"=enum."读数据保存请求2"} ("元素") cluster{"Data":string[], "State":T1} {"Data"=[], "State"=enum."读数据保存请求2"} ("元素") w3891 cluster{"Data":string[], "State":T1} {"Data"=[], "State"=enum."读扫码请求3"} ("元素") cluster{"Data":string[], "State":T1} {"Data"=[], "State"=enum."读扫码请求3"} ("元素") cluster{"Data":string[], "State":T1} {"Data"=[], "State"=enum."读扫码请求3"} ("元素") w3987 cluster{"Data":string[], "State":T1} {"Data"=[], "State"=enum."读数据保存请求3"} ("元素") cluster{"Data":string[], "State":T1} {"Data"=[], "State"=enum."读数据保存请求3"} ("元素") cluster{"Data":string[], "State":T1} {"Data"=[], "State"=enum."读数据保存请求3"} ("元素") w4105 cluster{"Data":string[], "State":T1} {"Data"=[], "State"=enum."看门狗"} ("元素") cluster{"Data":string[], "State":T1} {"Data"=[], "State"=enum."看门狗"} ("元素") cluster{"Data":string[], "State":T1} {"Data"=[], "State"=enum."读扫码请求"} ("元素") cluster{"Data":string[], "State":T1} {"Data"=[], "State"=enum."读扫码请求"} ("元素")] -> w3398
          tunnel: w3397 -> [_ _ _ _ w3557 _ _ _ w3706 _ _ _ _ _ _ w3819 _ _ _ w3965 _ _ _ w4046 _ _ _ w4213 _ _]
          tunnel: [FALSE FALSE FALSE FALSE FALSE FALSE FALSE FALSE FALSE FALSE FALSE TRUE FALSE FALSE FALSE FALSE FALSE FALSE FALSE FALSE FALSE FALSE FALSE FALSE FALSE FALSE FALSE FALSE FALSE FALSE] -> w3396
          tunnel: w3395 -> [_ _ _ _ _ _ _ w3675 _ _ w3722 w3734 _ _ w3791 _ _ _ w3931 _ _ _ _ _ _ _ _ _ _ _]
          tunnel: [T7 {"扫码超时1"="999", "数据保存超时1"="999", "扫码超时2"="999", "数据保存超时2"="999", "看门狗"="999", "扫码超时3"="999", "数据保存超时3"="999", "条码"="", "次数"=0} w3481 w3489 w3535 w3553 w3606 w3612 w3672 w3700 w3715 w3720 w3729 w3737 w3743 w3786 w3812 w3864 w3870 w3930 w3959 w3978 w3980 w4028 w4049 w4101 w4103 w4183 w4215 w4229 w4234] -> w3394
          tunnel: w3393 -> [_ w3481 w3489 w3535 w3554 w3606 w3612 w3672 w3701 w3715 w3720 w3729 w3737 w3743 w3786 w3813 w3864 w3871 w3930 w3960 w3978 w3980 w4028 w4051 w4101 w4103 w4183 w4216 w4229 w4235]
          frame "PLC通讯初始化", Default {
            w3428 = u16 0 items=["byte", "word", "Dword"] ("数据类型")
            w3424 = u8 132 items=["I/O (P)"=128, "Input (I)"=129, "Output (Q)"=130, "Bit Memory (M)"=131, "Data (DB)"=132, "Instance Data (DI)"=133, "Local Data (L)"=134, "Predecessor Local Data (VL)"=135] ("寄存器类型")
            w3435 = u16 0 items=["byte", "word", "Dword"] ("数据类型")
            w3431 = u8 132 items=["I/O (P)"=128, "Input (I)"=129, "Output (Q)"=130, "Bit Memory (M)"=131, "Data (DB)"=132, "Instance Data (DI)"=133, "Local Data (L)"=134, "Predecessor Local Data (VL)"=135] ("寄存器类型")
            w3455 = u8 0 items=["S7-1200.200.200SMART"=0, "S7-300"=2, "S7-400"=3] ("PLC 系列")
            n921 = Enqueue Element(queue=w3447, element=cluster{"Data":string[], "State":T1} {"Data"=["999"], "State"=enum."扫码回复"} ("元素")) -> (queue out=w3451:refnum<queue>, error out=w3450:errorcluster)  [unwired: 2 in, 1 out]
            n922 = call "S7_Open.vi"("IP 地址"="192.168.0.40", "PLC 系列"=w3455, "超时（MS）"=100) -> ("TCP"=w3419:refnum<k5>, "error out"=w3418:errorcluster)  [unwired: 10 in, 1 out]
            n923 = Enqueue Element(queue=w3451, element=cluster{"Data":string[], "State":T1} {"Data"=["999"], "State"=enum."数据保存回复"} ("元素"), error in (no error)=w3450) -> (queue out=w3446:refnum<queue>, error out=w3445:errorcluster)  [unwired: 1 in, 1 out]
            n924 = Unbundle By Name(w3418) -> ("status"=→"ST40通讯状态":bool)
            n925 = disable-structure shown="启用" {
              disable-tunnel: w3446 -> [w3460 w3466]
              disable-tunnel: w3445 -> [w3459 w3465]
              disable-tunnel: [w3458 w3466] -> w3439
              disable-tunnel: [w3457 w3465] -> w3438
              frame Disabled {
                n926 = Enqueue Element(queue=w3460, element=cluster{"Data":string[], "State":T1} {"Data"=["999"], "State"=enum."扫码回复2"} ("元素"), error in (no error)=w3459) -> (queue out=w3463:refnum<queue>, error out=w3464:errorcluster)  [unwired: 1 in, 1 out]
                n927 = Enqueue Element(queue=w3463, element=cluster{"Data":string[], "State":T1} {"Data"=["999"], "State"=enum."数据保存回复2"} ("元素"), error in (no error)=w3464) -> (queue out=w3458:refnum<queue>, error out=w3457:errorcluster)  [unwired: 1 in, 1 out]
              }
              frame Enabled {
              }
            }
            n928 = call "S7_Read.vi"("TCP"=w3419, "DB #"=u16 20, "读取长度"=u16 17, "寄存器类型"=w3431, "起始地址"=u32 24, "数据类型"=w3435, "error in"=w3418) -> ("TCP"=w3423:refnum<k5>, "数据"=w3436:u32[], "error out"=w3422:errorcluster)  [unwired: 5 in, 1 out]
            n929 = To Unsigned Word Integer(number=w3436) -> (unsigned 16bit integer=w3437:u16[])
            n930 = call "还原为字符串.vi"("输入数组"=w3437) -> ("字符串"=w3413:string)  [unwired: 9 in, 1 out]
            n931 = Match Pattern(string=w3413, regular expression=" " ("正则表达式")) -> (before substring=w3412:string)  [unwired: 1 in, 3 out]
            n932 = local write "401二维码"(w3412) -> ()
            n933 = Enqueue Element(queue=w3439, element=cluster{"Data":string[], "State":T1} {"Data"=["999"], "State"=enum."扫码回复3"} ("元素"), error in (no error)=w3438) -> (queue out=w3441:refnum<queue>, error out=w3440:errorcluster)  [unwired: 1 in, 1 out]
            n934 = disable-structure shown="禁用" {
              disable-tunnel: w3423 -> [w3470 w3480]
              disable-tunnel: w3422 -> [w3469 w3479]
              disable-tunnel: [w3468 w3480] -> w3421
              disable-tunnel: [w3467 w3479] -> w3420
              frame Disabled {
                w3475 = u16 0 items=["byte", "word", "Dword"] ("数据类型")
                w3471 = u8 132 items=["I/O (P)"=128, "Input (I)"=129, "Output (Q)"=130, "Bit Memory (M)"=131, "Data (DB)"=132, "Instance Data (DI)"=133, "Local Data (L)"=134, "Predecessor Local Data (VL)"=135] ("寄存器类型")
                n935 = call "S7_Read.vi"("TCP"=w3470, "DB #"=u16 20, "读取长度"=u16 17, "寄存器类型"=w3471, "起始地址"=u32 42, "数据类型"=w3475, "error in"=w3469) -> ("TCP"=w3468:refnum<k5>, "数据"=w3476:u32[], "error out"=w3467:errorcluster)  [unwired: 5 in, 1 out]
                n936 = To Unsigned Word Integer(number=w3476) -> (unsigned 16bit integer=w3477:u16[])
                n937 = call "还原为字符串.vi"("输入数组"=w3477) -> ("字符串"=w3478:string)  [unwired: 9 in, 1 out]
                n938 = local write "402二维码 2"(w3478) -> ()
              }
              frame Enabled {
              }
            }
            n939 = Enqueue Element(queue=w3441, element=cluster{"Data":string[], "State":T1} {"Data"=["999"], "State"=enum."数据保存回复3"} ("元素"), error in (no error)=w3440) -> ()  [unwired: 1 in, 3 out]
            n940 = call "S7_Read.vi"("TCP"=w3421, "DB #"=u16 20, "读取长度"=u16 17, "寄存器类型"=w3424, "起始地址"=u32 60, "数据类型"=w3428, "error in"=w3420) -> ("TCP"=w3417:refnum<k5>, "数据"=w3429:u32[], "error out"=w3416:errorcluster)  [unwired: 5 in, 1 out]
            n941 = To Unsigned Word Integer(number=w3429) -> (unsigned 16bit integer=w3430:u16[])
            n942 = call "还原为字符串.vi"("输入数组"=w3430) -> ("字符串"=w3410:string)  [unwired: 9 in, 1 out]
            n943 = Match Pattern(string=w3410, regular expression=" " ("正则表达式")) -> (before substring=w3409:string)  [unwired: 1 in, 3 out]
            n944 = local write "403二维码"(w3409) -> ()
          }
          frame "--------------" {
          }
          frame "读扫码请求" {
            w3516 = u16 0 items=["byte", "word", "Dword"] ("数据类型")
            w3518 = u8 132 items=["I/O (P)"=128, "Input (I)"=129, "Output (Q)"=130, "Bit Memory (M)"=131, "Data (DB)"=132, "Instance Data (DI)"=133, "Local Data (L)"=134, "Predecessor Local Data (VL)"=135] ("寄存器类型")
            n945 = call "S7_Read.vi"("TCP"=w3508, "DB #"=u16 20, "读取长度"=u16 1, "寄存器类型"=w3518, "起始地址"=u32 0, "数据类型"=w3516) -> ("TCP"=w3507:refnum<k5>, "数据"=w3513:u32[], "读取成功"=w3487:bool, "error out"=w3506:errorcluster)  [unwired: 6 in]
            n946 = Not(x=w3487) -> (.not. x?=w3486:bool)
            n947 = Index Array(array=w3513, index=0 ("索引")) -> (element=w3511:u32)
            n948 = local write "ST40通讯状态"(w3486) -> ()
            n949 = Number To Boolean Array(number=w3511) -> (Boolean array=w3510:bool[])
            n950 = Index Array(array=w3510, index=0 ("索引")) -> (element=w3495:bool)
            "ST401扫码请求" <- w3495
            n951 = Unbundle By Name(w3489) -> ("扫码超时1"=w3490:string)
            n952 = Not Equal?(x=w3490, y="999") -> (x != y?=w3492:bool)
            n953 = Not(x=w3492) -> (.not. x?=w3493:bool)
            n954 = call <vilib>:"Boolean Crossing PtByPt.vi"("direction"=enum16{"either", "false-true", "true-false"}."false-true", "input"=w3495) -> ("crossing"=w3502:bool)  [unwired: 1 in]
            n955 = call <vilib>:"Boolean Crossing PtByPt.vi"("direction"=enum16{"either", "false-true", "true-false"}."true-false", "input"=w3495) -> ("crossing"=w3501:bool)  [unwired: 1 in]
            n956 = call "已用时间9"("Reset"=w3493) -> ("Time has Elapsed"=w3494:bool)  [unwired: 11 in, 7 out]
            n957 = Insert Into Array(array=bool[] [] ("数组"), index=0 ("索引"), new element #1=w3502, new element #2=w3501) -> (w3498:bool[])
            n958 = Boolean Array To Number(Boolean array=w3498) -> (number=w3497:u32)
            n959 = case shown="真" w3494 {
              tunnel: w3488 -> [_ w3520]
              frame False {
              }
              frame True {
                n960 = Enqueue Element(queue=w3520, element=cluster{"Data":string[], "State":T1} {"Data"=["999"], "State"=enum."扫码回复"} ("元素"), timeout in ms (-1)=10 ("超时毫秒(-1)")) -> ()  [unwired: 1 in, 3 out]
              }
            }
            n961 = case shown="0, 默认" w3497 {
              tunnel: [cluster{"Data":string[], "State":T1} {"Data"=[], "State"=enum."读数据保存请求"} ("元素") w3524 w3526] -> w3496
              tunnel: w3488 -> [_ w3525 w3527]
              frame 0, Default {
              }
              frame 1 {
                w3524 = cluster{"Data":string[], "State":T1} {"Data"=[], "State"=enum."读二维码"} ("元素")
                n962 = Enqueue Element(queue=w3525, element=w3524, timeout in ms (-1)=10 ("超时毫秒(-1)")) -> ()  [unwired: 1 in, 3 out]
              }
              frame 2 {
                w3526 = cluster{"Data":string[], "State":T1} {"Data"=["999"], "State"=enum."扫码回复"} ("元素")
                n963 = Enqueue Element(queue=w3527, element=w3526, timeout in ms (-1)=10 ("超时毫秒(-1)")) -> ()  [unwired: 1 in, 3 out]
              }
            }
          }
          frame "读二维码" {
            w3544 = u16 0 items=["byte", "word", "Dword"] ("数据类型")
            w3540 = u8 132 items=["I/O (P)"=128, "Input (I)"=129, "Output (Q)"=130, "Bit Memory (M)"=131, "Data (DB)"=132, "Instance Data (DI)"=133, "Local Data (L)"=134, "Predecessor Local Data (VL)"=135] ("寄存器类型")
            n964 = call "S7_Read.vi"("TCP"=w3539, "DB #"=u16 20, "读取长度"=u16 17, "寄存器类型"=w3540, "起始地址"=u32 24, "数据类型"=w3544) -> ("TCP"=w3538:refnum<k5>, "数据"=w3545:u32[], "error out"=w3547:errorcluster)  [unwired: 6 in, 1 out]
            n965 = To Unsigned Word Integer(number=w3545) -> (unsigned 16bit integer=w3546:u16[])
            n966 = call "还原为字符串.vi"("error in (no error)"=w3547, "输入数组"=w3546) -> ("error out"=w3531:errorcluster, "字符串"=w3532:string)  [unwired: 8 in]
            n967 = Match Pattern(string=w3532, regular expression=" " ("正则表达式")) -> (before substring=w3529:string)  [unwired: 1 in, 3 out]
            n968 = flat-sequence {
              tunnel: w3531 -> [w3549]
              tunnel: [w3549] -> w3530
              tunnel: w3529 -> [w3548]
              tunnel: [w3552] -> w3534
              tunnel: w3530 -> [w3550]
              frame #0 {
                "401二维码" <- w3548
              }
              frame #1 {
                n969 = property on="ST401扫码请求(事件)" class="Bool (严格)"(error in=w3550, "Val(Sgnl)"=TRUE ("值(信号)")) -> (error out=w3552:errorcluster)  [unwired: 1 in, 1 out]
              }
            }
          }
          frame "扫码回复" {
            n970 = Array Size(array=w3557) -> (size(s)=w3556:i32)
            n971 = case shown="3, 默认" w3556 {
              tunnel: w3557 -> [w3587 w3596]
              tunnel: w3560 -> [w3574 w3597]
              tunnel: [w3565 w3599] -> w3559
              tunnel: [w3564 w3598] -> w3558
              tunnel: [w3563 w3595] -> w3555
              frame 3, Default {
                w3577 = u8 132 items=["I/O (P)"=128, "Input (I)"=129, "Output (Q)"=130, "Bit Memory (M)"=131, "Data (DB)"=132, "Instance Data (DI)"=133, "Local Data (L)"=134, "Predecessor Local Data (VL)"=135] ("寄存器类型")
                w3576 = u16 1 items=["byte", "word", "Dword"] ("数据类型")
                w3584 = u8 132 items=["I/O (P)"=128, "Input (I)"=129, "Output (Q)"=130, "Bit Memory (M)"=131, "Data (DB)"=132, "Instance Data (DI)"=133, "Local Data (L)"=134, "Predecessor Local Data (VL)"=135] ("寄存器类型")
                w3585 = u16 1 items=["byte", "word", "Dword"] ("数据类型")
                w3591 = u8 132 items=["I/O (P)"=128, "Input (I)"=129, "Output (Q)"=130, "Bit Memory (M)"=131, "Data (DB)"=132, "Instance Data (DI)"=133, "Local Data (L)"=134, "Predecessor Local Data (VL)"=135] ("寄存器类型")
                w3590 = u16 1 items=["byte", "word", "Dword"] ("数据类型")
                n972 = Index Array(array=w3587) -> (element #1=w3563:string, element #2=w3570:string, element #3=w3569:string)  [unwired: 3 in]
                n973 = Equal?(x=w3569, y="OK") -> (x = y?=w3567:bool)
                n974 = Decimal String To Number(string=w3570, default (0L)=u32 0 ("默认(0 I32)")) -> (number=w3571:u32)  [unwired: 1 in, 1 out]
                n975 = case shown="假" w3567 {
                  tunnel: [u32 2 ("写入数据") u32 1 ("写入数据")] -> w3566
                  frame False {
                  }
                  frame True {
                  }
                }
                n976 = call "S7_Write.vi"("TCP"=w3574, "寄存器类型"=w3591, "DB #"=u16 20, "写入地址"=u32 8, "数据类型"=w3590, "写入数据"=w3571) -> ("TCP"=w3581:refnum<k5>, "error out"=w3582:errorcluster)  [unwired: 7 in, 1 out]
                n977 = call "S7_Write.vi"("TCP"=w3581, "寄存器类型"=w3584, "DB #"=u16 20, "写入地址"=u32 10, "数据类型"=w3585, "写入数据"=w3566, "error in"=w3582) -> ("TCP"=w3573:refnum<k5>, "error out"=w3572:errorcluster)  [unwired: 6 in, 1 out]
                n978 = Decimal String To Number(string=w3563, default (0L)=u32 0 ("默认(0 I32)")) -> (number=w3580:u32)  [unwired: 1 in, 1 out]
                n979 = call "S7_Write.vi"("TCP"=w3573, "寄存器类型"=w3577, "DB #"=u16 20, "写入地址"=u32 2, "数据类型"=w3576, "写入数据"=w3580, "error in"=w3572) -> ("TCP"=w3565:refnum<k5>, "error out"=w3564:errorcluster)  [unwired: 6 in, 1 out]
              }
              frame 1 {
